vi "DefaultFromIni.vi"(8 "error in (no error)":errorcluster, 11 "PmuAnalysis in":refnum<class "PmuAnalysis.lvclass">) -> (0 "error out":errorcluster, 3 "PmuAnalysis out":refnum<class "PmuAnalysis.lvclass">)   [LabVIEW 2018, in "AnalysisPlugins.lvlib" / "PmuAnalysis.lvclass"]
uses:
  PmuAnalysis.lvclass
  <vilib>/Utility/config.llb/NI_LVConfig.lvlib
  <userlib>/NIST/BaseClasses/Object_class/BaseObject.lvclass
  FGen/MemberClasses/FunctionBaseClass/FunctionBase.lvclass
  <vilib>/Utility/error.llb/Error Cluster From Error Code.vi
  <vilib>/ErrorRing/Error Ring.xnode
  FitterBaseClass/FitterBase.lvclass
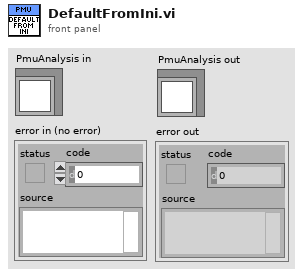
[diagram p1: front panel]
types:
  T1 = enum16{"SteadyState", "Modulation", "Ramp", "Step"}
  T2 = typedef "NI_LVConfig.lvlib/Config Data RefNum.ctl" = refnum<k1>
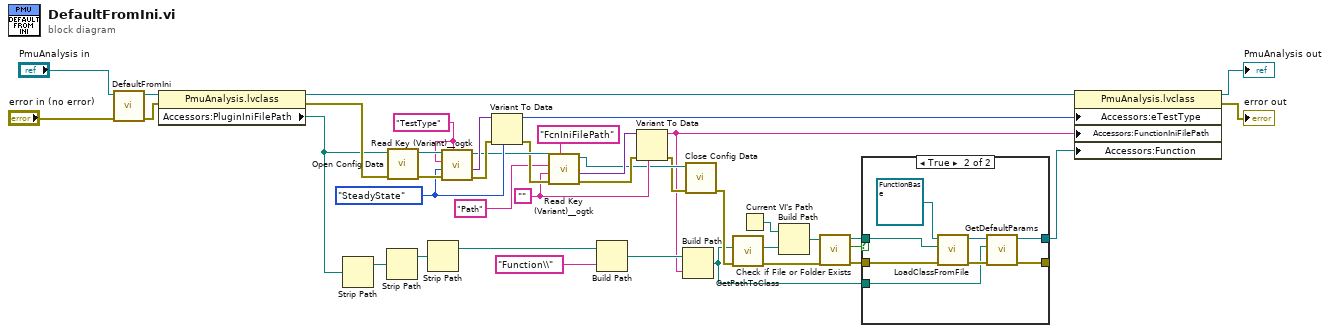
[diagram p0: block diagram]
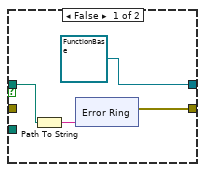
[diagram p2: hidden frame]
diagram:
  w22 = "" ("FunctionIniFilePath")
  w5 = "TestType" ("section")
  w29 = T1."SteadyState" ("eTestType")
  n1 = call-parent "DefaultFromIni.vi"("error in (no error)"="error in (no error)", "FitterBase in"="PmuAnalysis in") -> ("error out"=w41:errorcluster, "FitterBase out"=w38:refnum<class "PmuAnalysis.lvclass">)  [unwired: 8 in]
  n2 = property class="PmuAnalysis.lvclass"(reference=w38, error in=w41) -> (reference out=w36:refnum<class "PmuAnalysis.lvclass">, error out=w34:errorcluster, "Accessors:PluginIniFilePath"=w4:path)
  n3 = Strip Path(path=w4) -> (stripped path=w3:path)  [unwired: 1 out]
  n4 = Strip Path(path=w3) -> (stripped path=w2:path)  [unwired: 1 out]
  n5 = call <vilib>:"Open Config Data.vi"("error in (no error)"=w34, "configuration file path"=w4) -> ("error out"=w33:errorcluster, "refnum"=w32:T2)  [unwired: 7 in, 1 out]
  n6 = Strip Path(path=w2) -> (stripped path=w1:path)  [unwired: 1 out]
  n7 = call <userlib>:"Read Key (Variant)__ogtk.vi"("section"=w5, "error in (no error)"=w33, "type"=w29, "key (optional)"=w5, "refnum"=w32) -> ("error out"=w31:errorcluster, "key-value"=w30:variant, "refnum out"=w27:T2)  [unwired: 3 in, 1 out]
  n8 = Variant To Data(error in=w31, type=w29, Variant=w30) -> (data=w28:T1, error out=w26:errorcluster)
  n9 = call <userlib>:"Read Key (Variant)__ogtk.vi"("section"="FcnIniFilePath", "error in (no error)"=w26, "type"=w22, "key (optional)"="Path", "refnum"=w27) -> ("error out"=w23:errorcluster, "key-value"=w24:variant, "refnum out"=w21:T2)  [unwired: 3 in, 1 out]
  n10 = Build Path(base path=w1, name or relative path="Function\\") -> (appended path=w9:path)
  n11 = Variant To Data(error in=w23, type=w22, Variant=w24) -> (data=w7:string, error out=w20:errorcluster)
  n12 = Build Path(base path=w9, name or relative path=w7) -> (appended path=w8:path)
  n13 = call <vilib>:"Close Config Data.vi"("error in (no error)"=w20, "refnum"=w21) -> ("error out"=w19:errorcluster)  [unwired: 8 in, 1 out]
  n14 = call <userlib>:"GetPathToClass.vi"("error in (no error)"=w19, "configuration file path"=w8) -> ("error IO"=w15:errorcluster, "PathToClass"=w18:path)  [unwired: 8 in]
  n15 = Current VI's Path() -> (path=w17:path)
  n16 = Build Path(base path=w17, name or relative path=w18) -> (appended path=w16:path)
  n17 = call <vilib>:"Check if File or Folder Exists.vi"("error in (no error)"=w15, "path"=w16) -> ("error out"=w13:errorcluster, "file or folder exists?"=w12:bool, "dup path"=w14:path)  [unwired: 7 in]
  n18 = case shown="True" w12 {
    tunnel: [w44 w55] -> _
    tunnel: w13 -> [_ w60]
    tunnel: w14 -> [w43 w59]
    tunnel: [refnum<class "FunctionBase.lvclass"> refnum ("Functions.lvlib:FunctionBase.lvclass") w54] -> w11
    tunnel: w8 -> [_ w53]
    frame False {
      n19 = Path To String(path=w43) -> (string=w45:string)
      n20 = xnode "Error Ring"("parameter 0"=w45) -> ("error out"=w44:errorcluster)
    }
    frame True {
      n21 = call-dynamic "LoadClassFromFile.vi"("error in (no error)"=w60, "class path"=w59, "reference in"=refnum<class "FunctionBase.lvclass"> refnum ("Functions.lvlib:FunctionBase.lvclass")) -> ("error out"=w57:errorcluster, "reference out"=w56:refnum<class "FunctionBase.lvclass">)  [unwired: 7 in]
      n22 = call-dynamic "GetDefaultParams.vi"("error in (no error)"=w57, "Path"=w53, "FunctionBase in"=w56) -> ("error out"=w55:errorcluster, "FunctionBase out"=w54:refnum<class "FunctionBase.lvclass">)  [unwired: 7 in]
    }
  }
  n23 = property class="PmuAnalysis.lvclass"(reference=w36, "Accessors:eTestType"=w28, "Accessors:FunctionIniFilePath"=w7, "Accessors:Function"=w11) -> (reference out=→"PmuAnalysis out":refnum<class "PmuAnalysis.lvclass">, error out=→"error out":errorcluster)  [unwired: 1 in]
